vi "TestLights.vi"() -> ()   [LabVIEW 2012]
panel:
  in  "Boolean":bool
  in  "Slide":dbl(slide) scale=-1.0..1.0
  in  "stop":bool
  # "Lightsabers"
  # "Chopsticks"
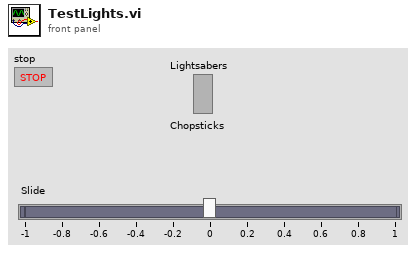
[diagram p1: front panel]
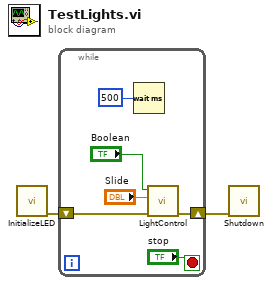
[diagram p0: block diagram]
diagram:
  n1 = call "InitializeLED.vi"() -> ("error out"=w1:errorcluster)  [unwired: 11 in]
  n2 = while {
    shift-right: [w4] -> w2
    shift-left: w1 -> [w8]
    stop <- "stop" stop-if-true
    n3 = Wait (ms)(milliseconds to wait=u32 500) -> ()  [unwired: 1 out]
    n4 = call "LightControl.vi"("error in (no error)"=w8, "X"="Slide", "Boolean"="Boolean") -> ("error out"=w4:errorcluster)  [unwired: 8 in]
  }
  n5 = call "Shutdown.vi"("error in (no error)"=w2) -> ()  [unwired: 10 in, 1 out]
